vi "gcodeTe2c.vi"() -> ()   [LabVIEW 2021]
panel:
  out "size(s)":i32[](array[numeric])
  out "array":dbl[][](array[numeric])
  out "X position":dbl
  out "Y position":dbl
  out "X":dbl
  out "Y":dbl
  out "Numeric":i32
  out "string in":string
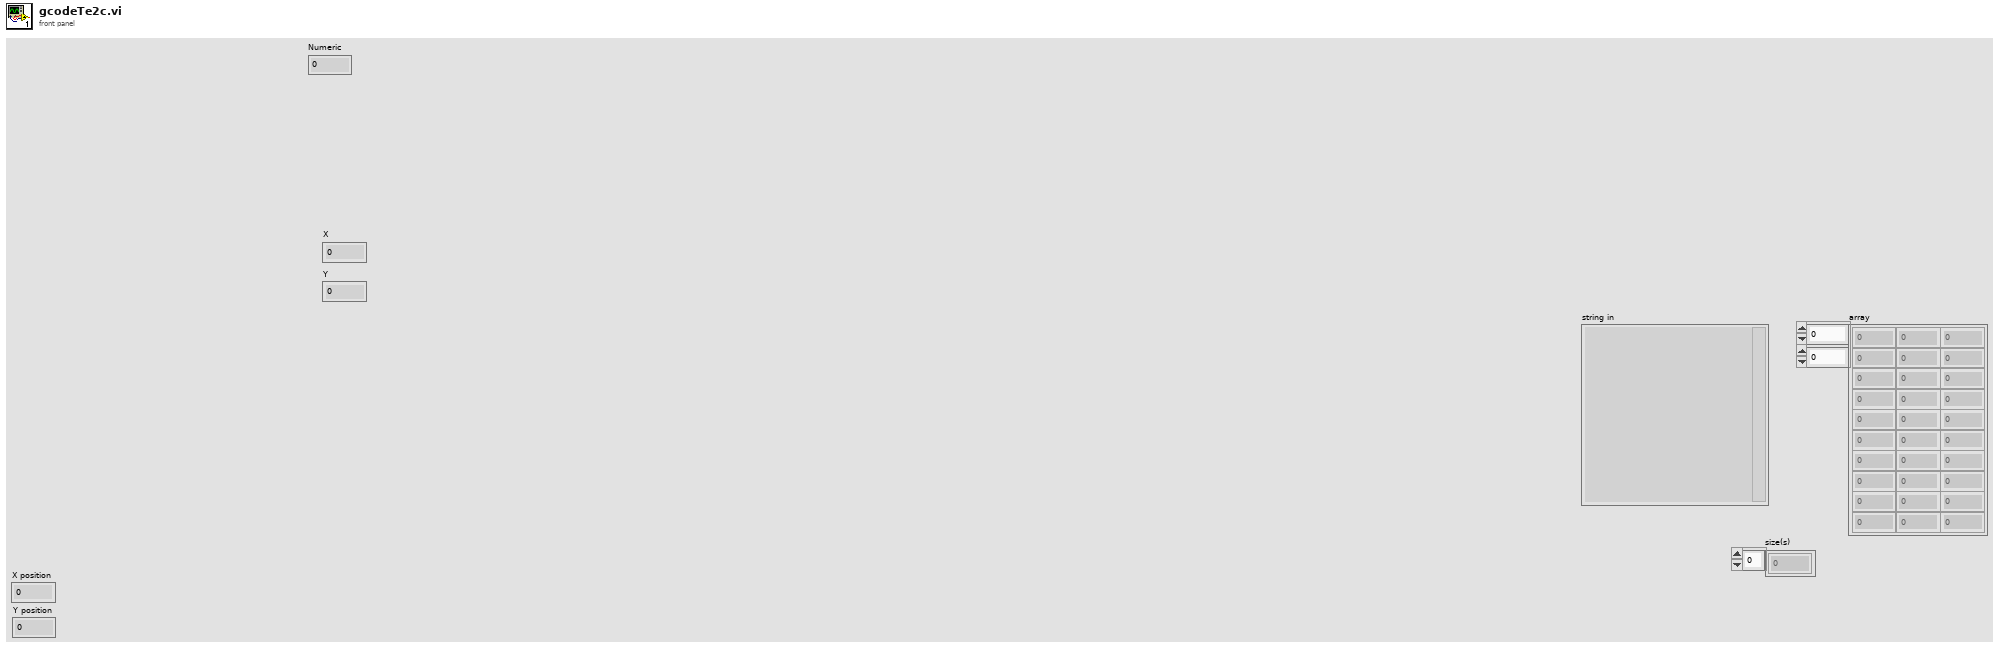
[diagram p1: front panel]
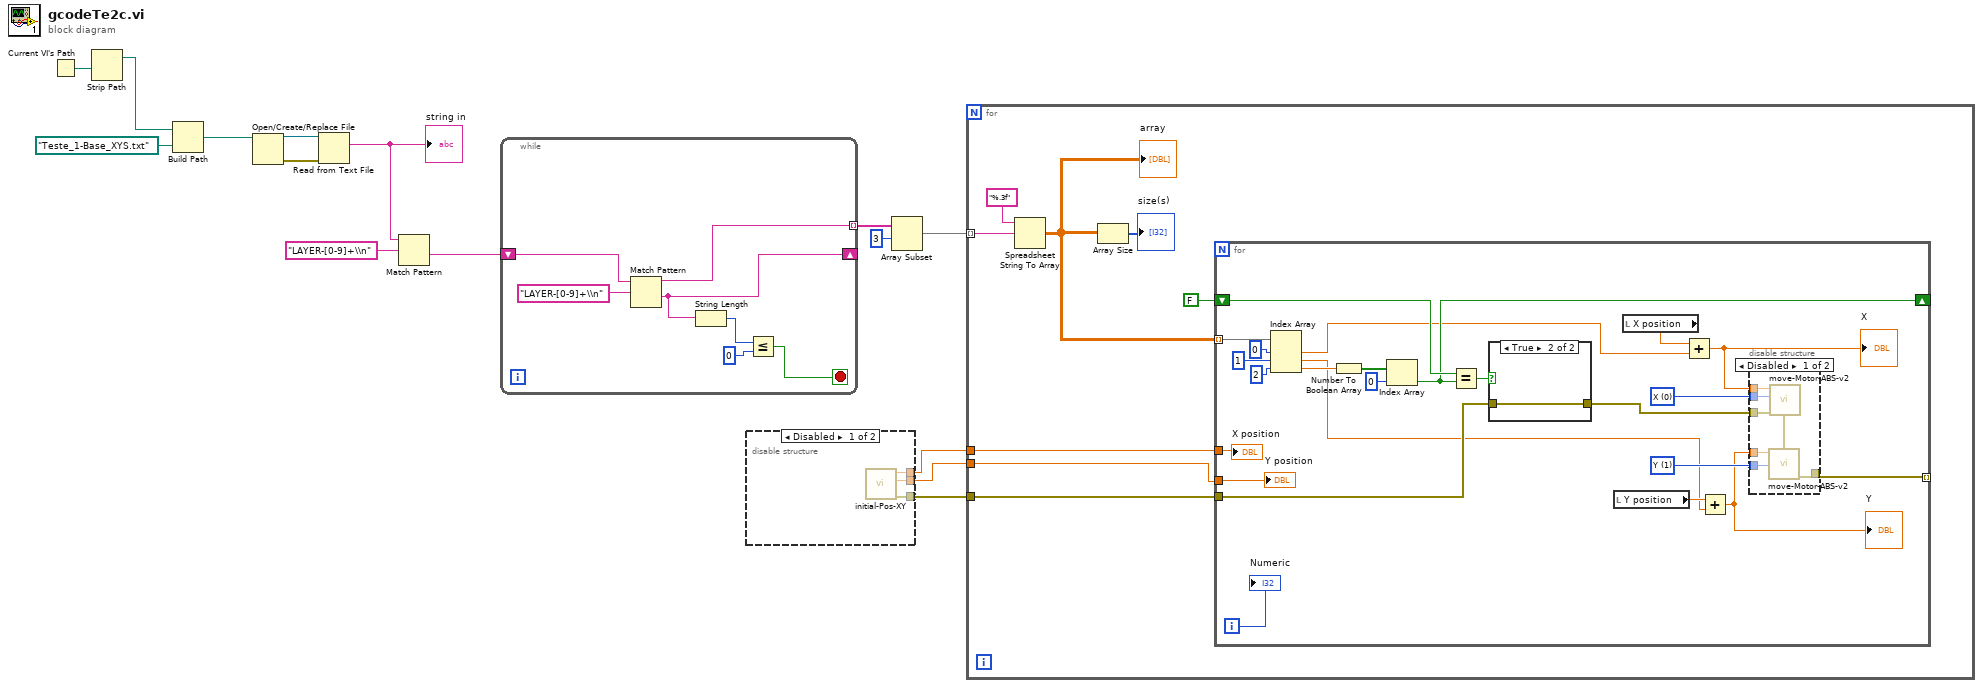
[diagram p0: block diagram]
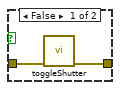
[diagram p4: hidden frame]
diagram:
  n1 = Current VI's Path() -> (path=w8:path)
  n2 = Strip Path(path=w8) -> (stripped path=w7:path)  [unwired: 1 out]
  n3 = Build Path(base path=w7, name or relative path=path "Teste_1-Base_XYS.txt" ("file path (use dialog)")) -> (appended path=w9:path)
  n4 = Open/Create/Replace File(file path (use dialog)=w9) -> (refnum out=w14:refnum<file>, error out=w15:errorcluster)  [unwired: 5 in, 1 out]
  n5 = Read from Text File(file (use dialog)=w14, error in=w15) -> (text=w13:string)  [unwired: 2 in, 3 out]
  "string in" <- w13
  n6 = Match Pattern(string=w13, regular expression="LAYER-[0-9]+\\n") -> (after substring=w11:string)  [unwired: 1 in, 3 out]
  n7 = while {
    shift-right: [w19] -> _
    shift-left: w11 -> [w21]
    tunnel: [w16] -> w6 mode=indexing
    stop <- w17 stop-if-true
    n8 = Match Pattern(string=w21, regular expression="LAYER-[0-9]+\\n") -> (before substring=w16:string, after substring=w19:string)  [unwired: 1 in, 2 out]
    n9 = String Length(string=w19) -> (length=w20:i32)
    n10 = Less Or Equal?(x=w20, y=0) -> (x <= y?=w17:bool)
  }
  n11 = disable-structure shown="Disabled" {
    disable-tunnel: [w25 _] -> w3
    disable-tunnel: [w24 _] -> w2
    disable-tunnel: [w23 _] -> w1
    frame Disabled {
      n12 = call "initial-Pos-XY.vi"() -> ("error out"=w25:errorcluster, "Y position"=w23:dbl, "X position"=w24:dbl)  [unwired: 9 in]
    }
    frame Enabled {
    }
  }
  n13 = Array Subset(array=w6, index=3) -> (w4:string[])  [unwired: 1 in]
  n14 = for {
    tunnel: w4 -> [w32] mode=indexing
    tunnel: w3 -> [w30]
    tunnel: w2 -> [w29]
    tunnel: w1 -> [w28]
    n15 = Spreadsheet String To Array(format string="%.3f", spreadsheet string=w32) -> (array=w33:dbl[][])  [unwired: 2 in]
    "array" <- w33
    n16 = Array Size(array=w33) -> (size(s)=→"size(s)":i32[])
    n17 = for {
      tunnel: w33 -> [w57] mode=indexing
      shift-right: [w48] -> _
      shift-left: FALSE -> [w50]
      tunnel: w30 -> [w47]
      tunnel: w29 -> [w42]
      tunnel: w28 -> [w41]
      tunnel: [w43] -> _ mode=indexing
      i -> [w34]
      w44 = u16 1 items=["X", "Y", "Z"] ("Axis")
      w45 = u16 0 items=["X", "Y", "Z"] ("Axis")
      n18 = Index Array(array=w57, index #1=0 ("index"), index #2=1 ("index"), index #3=2 ("index")) -> (element #1=w36:dbl, element #2=w35:dbl, element #3=w53:dbl)
      n19 = Number To Boolean Array(number=w53) -> (Boolean array=w52:bool[])
      n20 = Index Array(array=w52, index=0) -> (element=w48:bool)
      n21 = Equal?(x=w50, y=w48) -> (x = y?=w49:bool)
      n22 = case shown="True" w49 {
        tunnel: w47 -> [w66 w67]
        tunnel: [w65 w67] -> w46
        frame False {
          n23 = call "toggleShutter.vi"("Error In"=w66) -> ("error out"=w65:errorcluster)  [unwired: 9 in]
        }
        frame True {
        }
      }
      n24 = local read "Y position"() -> (w38:dbl)
      n25 = local read "X position"() -> (w40:dbl)
      n26 = Add(x=w40, y=w36) -> (x+y=w39:dbl)
      "X" <- w39
      n27 = Add(x=w38, y=w35) -> (x+y=w37:dbl)
      "Y" <- w37
      n28 = disable-structure shown="Disabled" {
        disable-tunnel: w46 -> [w64 _]
        disable-tunnel: w45 -> [w63 _]
        disable-tunnel: w44 -> [w61 _]
        disable-tunnel: [w60 _] -> w43
        disable-tunnel: w39 -> [w59 _]
        disable-tunnel: w37 -> [w58 _]
        frame Disabled {
          n29 = call "move-Motor-ABS-v2.vi"("error in"=w64, "Axis"=w63, "Distance (um)"=w59) -> ("error out"=w62:errorcluster)  [unwired: 8 in]
          n30 = call "move-Motor-ABS-v2.vi"("error in"=w62, "Axis"=w61, "Distance (um)"=w58) -> ("error out"=w60:errorcluster)  [unwired: 8 in]
        }
        frame Enabled {
        }
      }
      "X position" <- w42
      "Y position" <- w41
      "Numeric" <- w34
    }
  }
